vi "MeasureBreakdown.vi"(1 "Microsites":refnum<k24>, 2 "Junction Name":string, 7 ".NET Refnum":refnum<k24>, 9 "Function":string, 12 "appended path":path, 13 "new file path (Not A Path if cancelled)":path, 14 "UiDefinition":T1) -> (15 "error out":errorcluster)   [LabVIEW 2020]
uses:
  UIReferences.ctl
  C:/Users/User/Desktop/Automation/CurrentVersion/LabviewDXFViewer/bin/Release/LabviewDXFViewer.exe
  LabviewDXFViewer/bin/Release/LabviewDXFViewer.exe
  <vilib>/Utility/file.llb/Write Delimited Spreadsheet (DBL).vi
  <vilib>/Utility/file.llb/Write Delimited Spreadsheet (string).vi
panel:
  in  "CurrentPositionIndex":i32
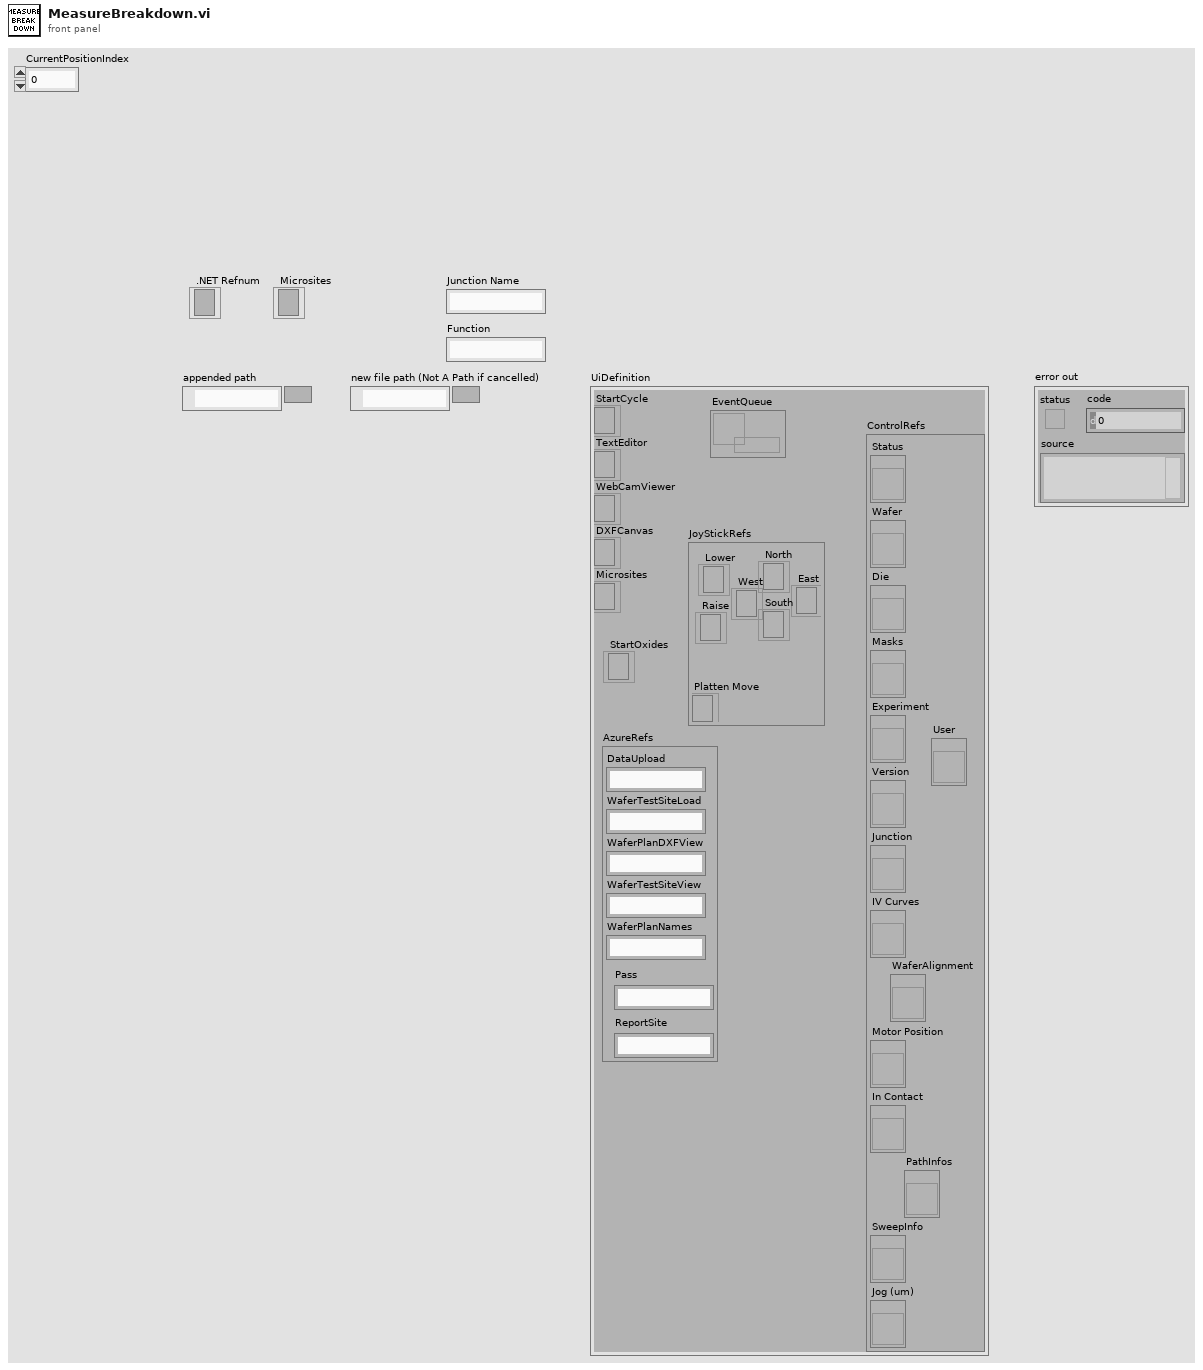
[diagram p1: front panel]
types:
  T1 = typedef "UIReferences.ctl" = cluster{"StartCycle":refnum<k24>, "TextEditor":refnum<k24>, "WebCamViewer":refnum<k24>, "DXFCanvas":refnum<k24>, "Microsites":refnum<k24>, "JoyStickRefs":cluster{"North":refnum<k24>, "Lower":refnum<k24>, "Raise":refnum<k24>, "Platten Move":refnum<k24>, "West":refnum<k24>, "East":refnum<k24>, "South":refnum<k24>}, "AzureRefs":cluster{"DataUpload":string, "WaferTestSiteLoad":string, "WaferPlanDXFView":string, "WaferTestSiteView":string, "WaferPlanNames":string, "Pass":string, "ReportSite":string}, "ControlRefs":cluster{"Status":refnum<vi>, "Wafer":refnum<vi>, "Die":refnum<vi>, "Masks":refnum<vi>, "Experiment":refnum<vi>, "Version":refnum<vi>, "Junction":refnum<vi>, "IV Curves":refnum<vi>, "Motor Position":refnum<vi>, "In Contact":refnum<vi>, "SweepInfo":refnum<vi>, "Jog (um)":refnum<vi>, "PathInfos":refnum<vi>, "User":refnum<vi>, "WaferAlignment":refnum<vi>}, "EventQueue":refnum<queue>, "StartOxides":refnum<k24>}
  T2 = typedef "CapacitanceInfos.ctl" = cluster{"Conductance":dbl, "CapacitanceIV":dbl, "Intercept":dbl, "CapacitanceSW":dbl, "Sum":dbl, "CapacitanceInfos":T3[], "CapacitancePhase":dbl, "dC/dV":dbl, "Function":string, "OtherInfo":dbl[][]}
  T3 = typedef "CapacitanceRecord.ctl" = cluster{"Freq":dbl, "Vpp":dbl, "PhaseS":dbl, "Irms":dbl, "PhaseC":dbl, "Theta":dbl, "VDrive":dbl, "Capacitance":dbl, "Other":dbl}
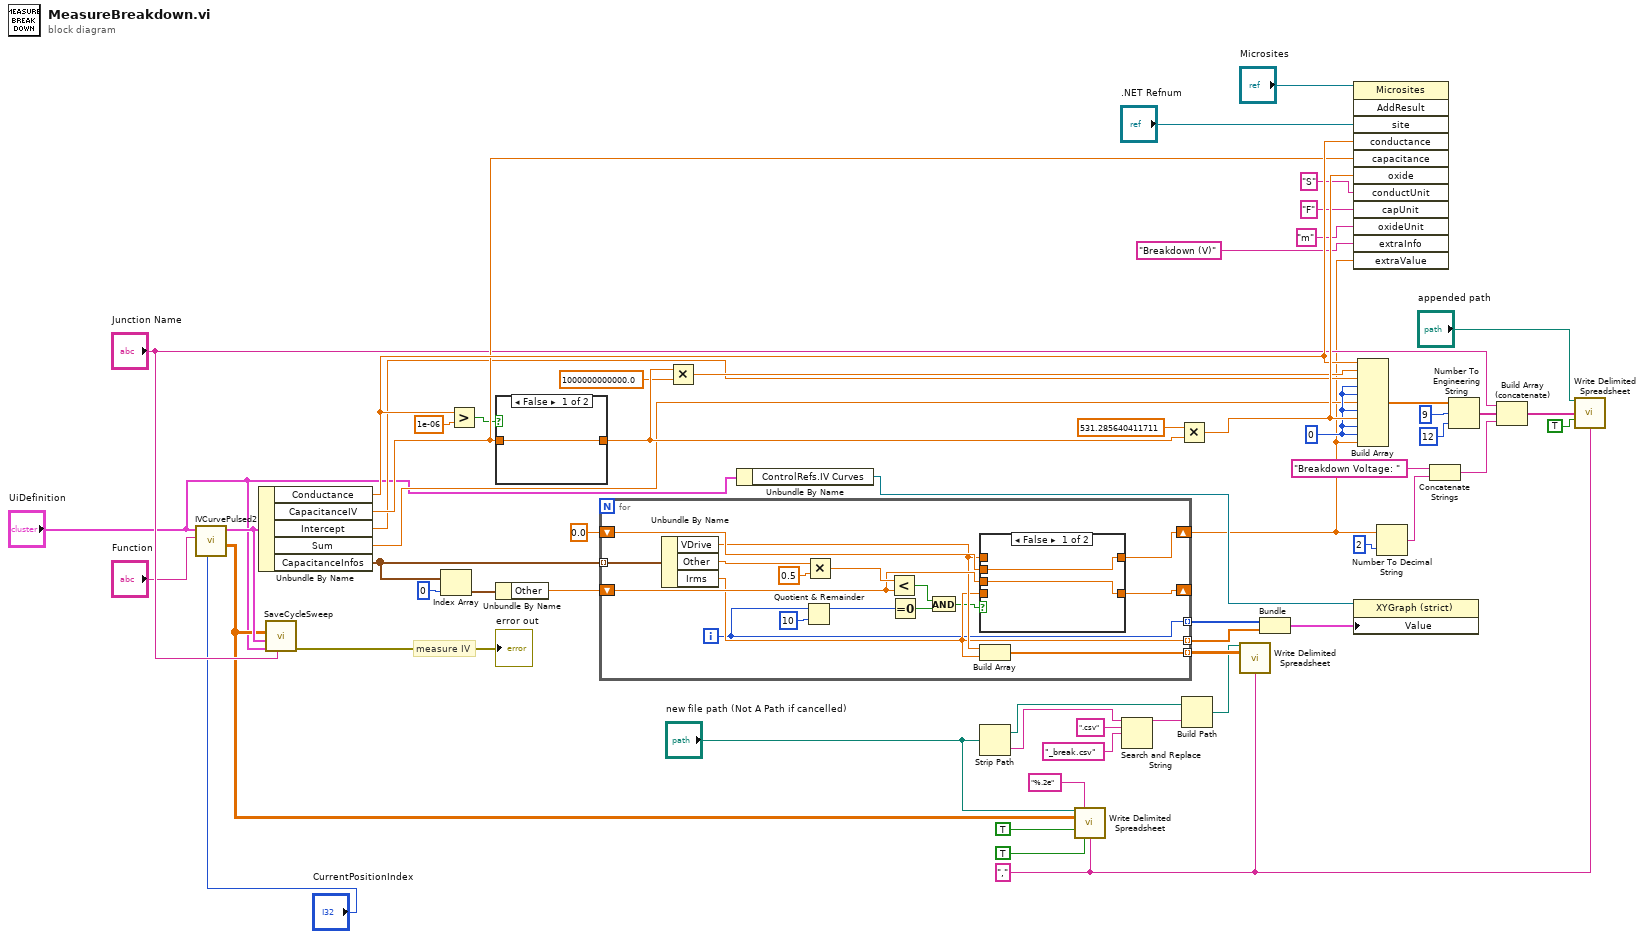
[diagram p0: block diagram]
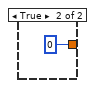
[diagram p3: hidden frame]
diagram:
  w18 = "," ("delimiter (\\t)")
  w48 = 0
  # "measure IV"
  n1 = call "IVCurvePulsed2.vi"("CurrentPositionIndex"="CurrentPositionIndex", "Program"="Function", "UiDefinition"="UiDefinition") -> ("appended array"=w27:dbl[][], "InfoCluster"=w40:T2)  [unwired: 7 in]
  n2 = Unbundle By Name(w40) -> ("Conductance"=w47:dbl, "CapacitanceIV"=w46:dbl, "Intercept"=w30:dbl, "Sum"=w31:dbl, "CapacitanceInfos"=w51:T3[])
  n3 = call "SaveCycleSweep.vi"("JunctionName"="Junction Name", "UiDefinition 2"="UiDefinition", "InfoCluster"=w40, "appended array"=w27) -> ("error out"=→"error out":errorcluster)  [unwired: 7 in]
  n4 = Index Array(array=w51, index=0) -> (element=w53:T3)
  n5 = Greater?(x=w47, y=1e-06) -> (0:w34:bool)
  n6 = case shown="False" w34 {
    tunnel: [w59 0] -> w57
    tunnel: w46 -> [w59 _]
    frame False {
    }
    frame True {
    }
  }
  n7 = Unbundle By Name(w53) -> ("Other"=w54:dbl)
  n8 = for {
    tunnel: w51 -> [w77] mode=indexing
    tunnel: [w65] -> w49 mode=indexing
    tunnel: [w66] -> w50 mode=indexing
    shift-right: [w70] -> _
    shift-left: w54 -> [w71]
    shift-right: [w75] -> w3
    shift-left: 0.0 ("Vpp") -> [w74]
    tunnel: [w67] -> w20 mode=indexing
    i -> [w65]
    n9 = Unbundle By Name(w77) -> ("VDrive"=w68:dbl, "Other"=w69:dbl, "Irms"=w66:dbl)
    n10 = Quotient & Remainder(x=w65, y=10) -> (x-y*floor(x/y)=w61:i32)  [unwired: 1 out]
    n11 = Multiply(x=w69, y=0.5) -> (x*y=w73:dbl)
    n12 = Less?(x=w73, y=w71) -> (x < y?=w76:bool)
    n13 = Equal To 0?(x=w61) -> (x = 0?=w62:bool)
    n14 = And(x=w76, y=w62) -> (x .and. y?=w63:bool)
    n15 = case shown="False" w63 {
      tunnel: w68 -> [_ w81]
      tunnel: [w79 w81] -> w75
      tunnel: w74 -> [w79 _]
      tunnel: [w78 w80] -> w70
      tunnel: w71 -> [w78 _]
      tunnel: w66 -> [_ w80]
      frame False {
      }
      frame True {
      }
    }
    n16 = Build Array(w68, w66) -> (w67:dbl[])
  }
  n17 = Multiply(x=w57, y=1000000000000.0) -> (x*y=w32:dbl)
  n18 = Unbundle By Name("UiDefinition") -> ("ControlRefs.IV Curves"=w9:refnum<vi>)
  n19 = Strip Path(path="new file path (Not A Path if cancelled)") -> (stripped path=w12:path, name=w16:string)
  n20 = call-poly <vilib>:"Write Delimited Spreadsheet.vi"("file path (dialog if empty)"="new file path (Not A Path if cancelled)", "format (%.3f)"="%.2e", "2D data"=w27, "append to file? (new file:F)"=TRUE, "transpose? (no:F)"=TRUE, "delimiter (\\t)"=w18) -> ()  [unwired: 8 in, 2 out]
  n21 = Search and Replace String(input string=w16, search string=".csv", replace string="_break.csv" ("replace string (\"\")")) -> (result string=w13:string)  [unwired: 5 in, 3 out]
  n22 = Multiply(x=531.285640411711, y=w57) -> (x*y=w58:dbl)
  n23 = Build Path(base path=w12, name or relative path=w13) -> (appended path=w11:path)
  n24 = call-poly <vilib>:"Write Delimited Spreadsheet.vi"("file path (dialog if empty)"=w11, "2D data"=w20, "delimiter (\\t)"=w18) -> ()  [unwired: 11 in, 2 out]
  n25 = Bundle(w49, w50) -> (w8:cluster{i32[], dbl[]})  [unwired: 1 in]
  n26 = invoke class="Microsites" method="AddResult"(reference="Microsites", "site"=".NET Refnum", "conductance"=w47, "capacitance"=w46, "oxide"=w58, "conductUnit"="S", "capUnit"="F", "oxideUnit"="m" ("interceptUnit"), "extraInfo"="Breakdown (V)", "extraValue"=w3) -> ()  [unwired: 2 in, 12 out]
  n27 = property class="XYGraph (strict)"(reference=w9, "Value"=w8) -> ()  [unwired: 1 in, 2 out]
  n28 = Build Array(w47, w32, w30, w48, w48, w31, w48, w58, w48, w48, w3) -> (w29:dbl[])
  n29 = Number To Decimal String(number=w3, width (-)=i16 2) -> (decimal integer string=w7:string)
  n30 = Concatenate Strings("Breakdown Voltage: ", w7) -> (w4:string)
  n31 = Number To Engineering String(2:i16 12 ("precision (6)"), 3:i16 9 ("width (-)"), 4:w29) -> (0:w21:string[])  [unwired: 1 in]
  n32 = Build Array (concatenate)("Junction Name", w21, w4) -> (w23:string[])
  n33 = call-poly <vilib>:"Write Delimited Spreadsheet.vi"("file path (dialog if empty)"="appended path", "1D data"=w23, "append to file? (new file:F)"=TRUE, "delimiter (\\t)"=w18) -> ()  [unwired: 10 in, 2 out]
